vi "Without Test Prefix.vi"(8 "error in (no error)":errorcluster, 11 "Parametrized Test Case Test Double in":refnum<class "Parametrized Test Case Test Double.lvclass">) -> (0 "error out":errorcluster, 3 "Parametrized Test Case Test Double out":refnum<class "Parametrized Test Case Test Double.lvclass">)   [LabVIEW 2020, in "Parametrized Test Case Test Double.lvclass"]
uses:
  Parametrized Test Case Test Double.lvclass
  Parametrized Test Case Test Double.lvclass/Parametrized Test Case Test Double.ctl
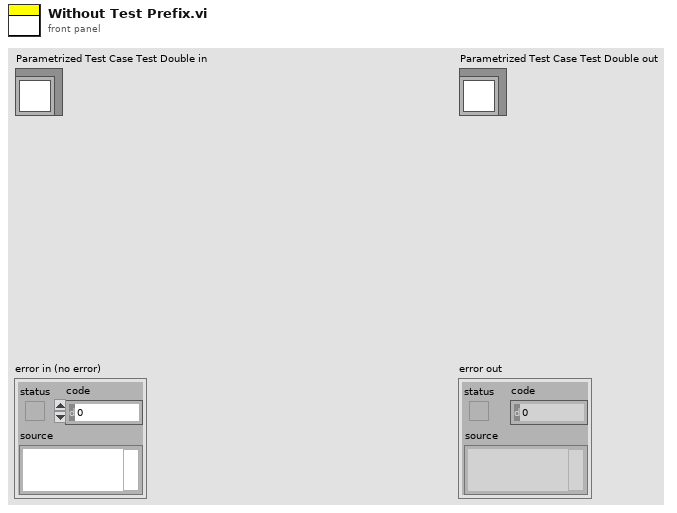
[diagram p1: front panel]
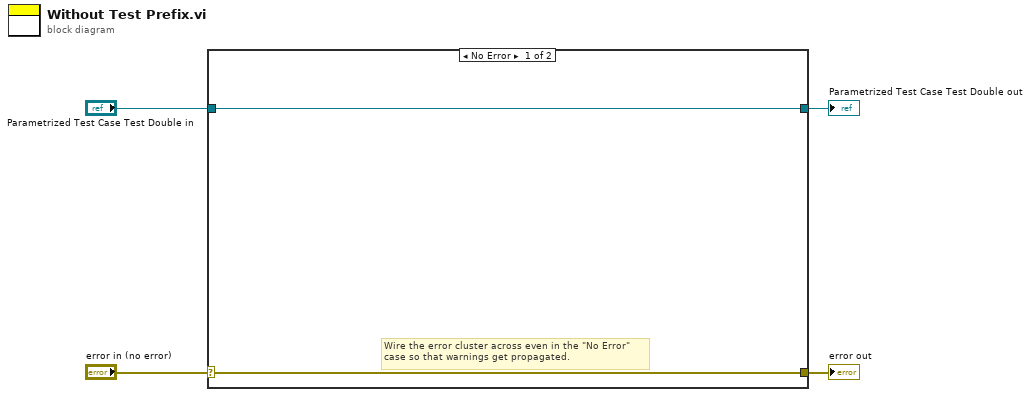
[diagram p0: block diagram]
diagram:
  n1 = case shown="No Error" "error in (no error)" {
    selector: "error in (no error)" -> [w5 w8]
    tunnel: [w5 w8] -> w3
    tunnel: [w6 w7] -> w1
    tunnel: "Parametrized Test Case Test Double in" -> [w6 w7]
    frame No Error {
      # "Wire the error cluster across even in the \"No Error\"\ncase so that warnings get propagated."
    }
    frame Error {
    }
  }
  "error out" <- w3
  "Parametrized Test Case Test Double out" <- w1
